vi "init.vi"(8 "error in":errorcluster, 10 "TBM module configuration in":refnum<class "TBM module configuration.lvclass">, 11 "dds runtime in":refnum<class "dds runtime.lvclass">) -> (0 "error out":errorcluster, 1 "data allocations":T1, 2 "execution settings":T4, 3 "dds runtime out":refnum<class "dds runtime.lvclass">)   [LabVIEW 2020, in "DDS runtime.lvclass"]
doc: "Provides an interface for initializing a module at runtime. While this interface performs no operations, a child should provide an override which may open any necessary references or sessions, allocate necessary memory, and perform any final configuration validataion before providing the full configuration <b>execution data</b> to the calling process."
uses:
  dds runtime.lvclass
  <vilib>/NI/Tag Bus Module Framework/module configuration/TBM module configuration.lvclass
  <vilib>/NI/Tag Bus Module Framework/runtime/execution settings.ctl
  <vilib>/NI/Tag Bus Module Framework/channel/data tables.ctl
  <vilib>/NI/Tag Bus/dictionary/data dictionary.lvclass
  <vilib>/NI/Tag Bus/dictionary table pair.ctl
  <vilib>/NI/Tag Bus/table/data table.ctl
  configuration/dds configuration.lvclass
  configuration/dds configuration.lvclass/dds configuration.ctl
  <vilib>/NI/Tag Bus Module Framework/channel/TBM channel.lvclass/TBM channel.ctl
  dds runtime.lvclass/dds runtime.ctl
  <vilib>/NI/Tag Bus/tag/Data Type.ctl
  <vilib>/NI/Tag Bus/tag/tag descriptor.lvclass/tag descriptor.ctl
  <vilib>/RTI DDS Toolkit/VIs/AdvancedCreateReader_NumDbl.vi
  <vilib>/RTI DDS Toolkit/VIs/AdvancedCreateReader_NumSgl.vi
  <vilib>/RTI DDS Toolkit/VIs/AdvancedCreateReader_NumI64.vi
  <vilib>/RTI DDS Toolkit/VIs/AdvancedCreateReader_NumI32.vi
  <vilib>/RTI DDS Toolkit/VIs/AdvancedCreateReader_NumI16.vi
  <vilib>/RTI DDS Toolkit/VIs/AdvancedCreateReader_NumI8.vi
  <vilib>/RTI DDS Toolkit/VIs/AdvancedCreateReader_NumU64.vi
  <vilib>/RTI DDS Toolkit/VIs/AdvancedCreateReader_NumU32.vi
  <vilib>/RTI DDS Toolkit/VIs/AdvancedCreateReader_NumU16.vi
  <vilib>/RTI DDS Toolkit/VIs/AdvancedCreateReader_NumU8.vi
  <vilib>/RTI DDS Toolkit/VIs/AdvancedCreateReader_Bool.vi
  <vilib>/RTI DDS Toolkit/VIs/AdvancedCreateReader_String.vi
  <vilib>/RTI DDS Toolkit/VIs/AdvancedCreateWriter_NumDbl.vi
  <vilib>/RTI DDS Toolkit/VIs/AdvancedCreateWriter_NumSgl.vi
  <vilib>/RTI DDS Toolkit/VIs/AdvancedCreateWriter_NumI64.vi
  <vilib>/RTI DDS Toolkit/VIs/AdvancedCreateWriter_NumI32.vi
  <vilib>/RTI DDS Toolkit/VIs/AdvancedCreateWriter_NumI16.vi
  <vilib>/RTI DDS Toolkit/VIs/AdvancedCreateWriter_NumI8.vi
  <vilib>/RTI DDS Toolkit/VIs/AdvancedCreateWriter_NumU64.vi
  <vilib>/RTI DDS Toolkit/VIs/AdvancedCreateWriter_NumU32.vi
  <vilib>/RTI DDS Toolkit/VIs/AdvancedCreateWriter_NumU16.vi
  <vilib>/RTI DDS Toolkit/VIs/AdvancedCreateWriter_NumU8.vi
  <vilib>/RTI DDS Toolkit/VIs/AdvancedCreateWriter_Bool.vi
  <vilib>/RTI DDS Toolkit/VIs/AdvancedCreateWriter_String.vi
  <vilib>/NI/Tag Bus Module Framework/channel/TBM channel.lvclass
  C:/Program Files (x86)/National Instruments/LabVIEW 2020/vi.lib/NI/Tag Bus/tag/tag descriptor.lvclass
  <vilib>/NI/Tag Bus Module Framework/runtime/TBM module execution interface.lvclass
  <vilib>/NI/Tag Bus/tag/tag descriptor.lvclass
  <vilib>/RTI DDS Toolkit/Library/LVDDS_library.lvlib
  <vilib>/NI/Tag Bus/tag bus.lvlib
  <vilib>/NI/Tag Bus/table/data table.lvlib
panel:
  out "Numeric":i32
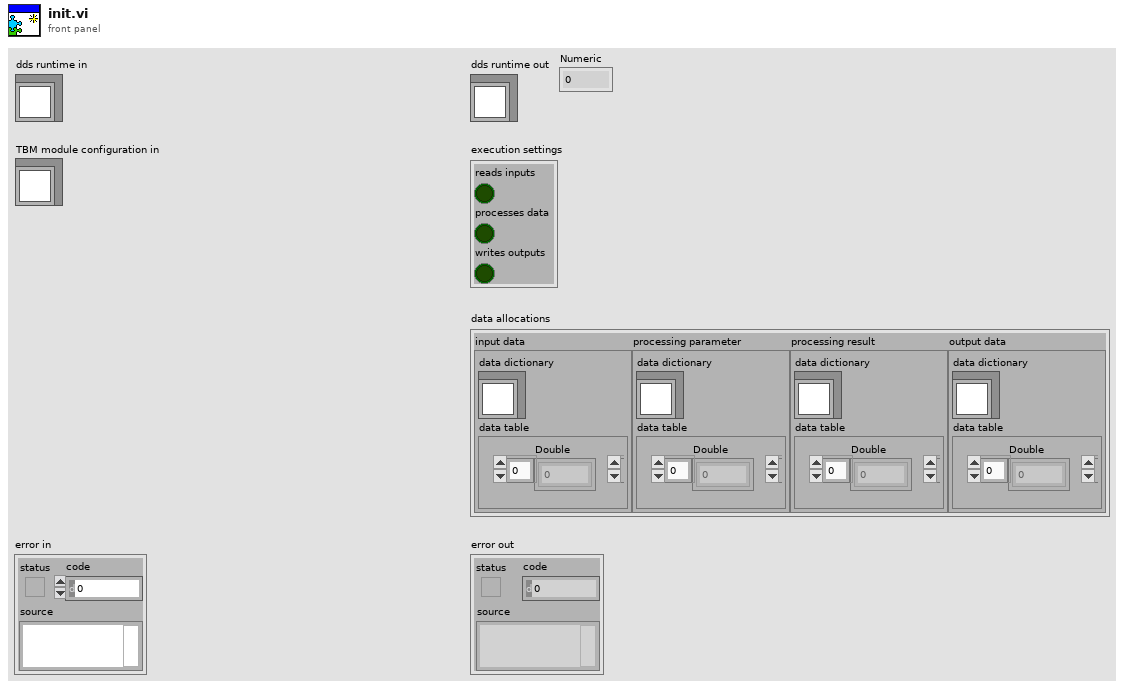
[diagram p1: front panel]
types:
  T1 = typedef "TBM channel.lvclass/data tables.ctl" = cluster{"input data":T2, "processing parameter":T2, "processing result":T2, "output data":T2}
  T2 = typedef "tag bus.lvlib/dictionary table pair.ctl" = cluster{"data dictionary":refnum<class "data dictionary.lvclass">, "data table":T3}
  T3 = typedef "tag bus.lvlib/data table.lvlib/data table.ctl" = cluster{"Double":dbl[], "Single":sgl[], "I64":i64[], "I32":i32[], "I16":i16[], "I8":i8[], "U64":u64[], "U32":u32[], "U16":u16[], "U8":u8[], "Boolean":bool[], "String":string[], "Array of Double":cluster{"DBL Array":dbl[]}[], "Array of Single":cluster{"SGL Array":sgl[]}[], "Array of I64":cluster{"I64 Array":i64[]}[], "Array of I32":cluster{"I32 Array":i32[]}[], "Array of I16":cluster{"I16 Array":i16[]}[], "Array of I8":cluster{"I8 Array":i8[]}[], "Array of U64":cluster{"U64 Array":u64[]}[], "Array of U32":cluster{"U32 Array":u32[]}[], "Array of U16":cluster{"U16 Array":u16[]}[], "Array of U8":cluster{"U8 Array":u8[]}[], "Array of Boolean":cluster{"Boolean Array":bool[]}[], "Array of String":cluster{"String Array":string[]}[]}
  T4 = typedef "TBM module execution interface.lvclass/execution settings.ctl" = cluster{"reads inputs":bool, "processes data":bool, "writes outputs":bool}
  T5 = typedef "tag bus.lvlib/tag descriptor.lvclass/Data Type.ctl" = enum16{"Double", "Single", "I64", "I32", "I16", "I8", "U64", "U32", "U16", "U8", "Boolean", "String", "Array of Double", "Array of Single", "Array of I64", "Array of I32", "Array of I16", "Array of I8", "Array of U64", "Array of U32", "Array of U16", "Array of U8", "Array of Boolean", "Array of String"}
  T6 = cluster{"index":i32, "data type":T5, "ref num":u64, "new samples only":bool, "query condition":string}
  T7 = cluster{"index":i32, "data type":T5, "ref num":u64}
  T8 = typedef "DDS configuration.lvclass/Line.ctl" = cluster{"channel":refnum<class "TBM channel.lvclass">, "DDS topic":string, "DDS Domain":u32, "advanced configuration":T9}
  T9 = typedef "LVDDS_library.lvlib/RTI DDS Advanced Reader Configuration.ctl" = cluster{"typeName":string, "keyName":string, "domainParticipantQoSProfile":string, "dataReaderQoSProfile":string, "forceArrayMapping?":bool, "forceExclusiveReader?":bool, "forceRead? (only ExclusiveReader)":bool, "forceUnboundedString?":bool}
  T10 = typedef "TBM channel.lvclass/channel classification.ctl" = enum16{"input data", "output data", "processing parameter", "processing result"}
  T11 = cluster{"index":i32, "data type":T5, "ref num":u64, "new samples only":bool, "query condition":string}[]
  T12 = cluster{"index":i32, "data type":T5, "ref num":u64}[]
  T13 = typedef "LVDDS_library.lvlib/RTI DDS Advanced Writer Configuration.ctl" = cluster{"typeName":string, "keyName":string, "domainParticipantQoSProfile":string, "dataWriterQoSProfile":string, "forceArrayMapping?":bool, "forceUnboundedString?":bool}
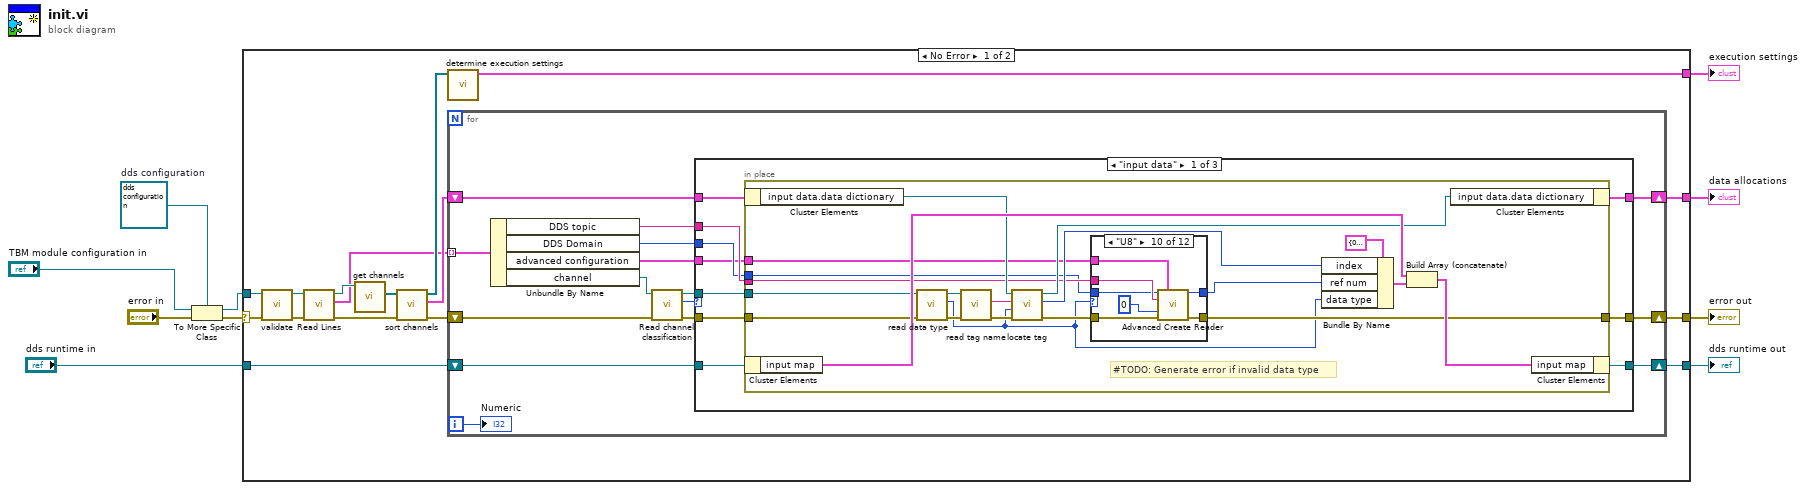
[diagram p0: block diagram]
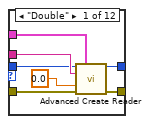
[diagram p2: hidden frame]
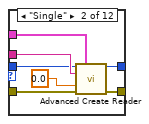
[diagram p3: hidden frame]
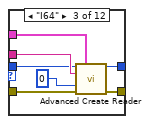
[diagram p4: hidden frame]
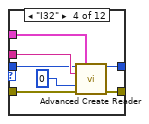
[diagram p5: hidden frame]
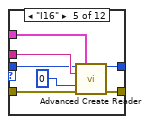
[diagram p6: hidden frame]
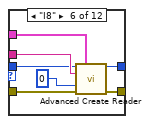
[diagram p7: hidden frame]
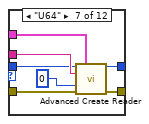
[diagram p8: hidden frame]
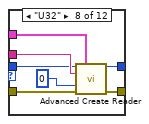
[diagram p9: hidden frame]
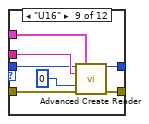
[diagram p10: hidden frame]
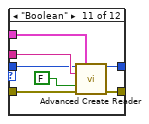
[diagram p11: hidden frame]
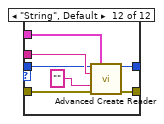
[diagram p12: hidden frame]
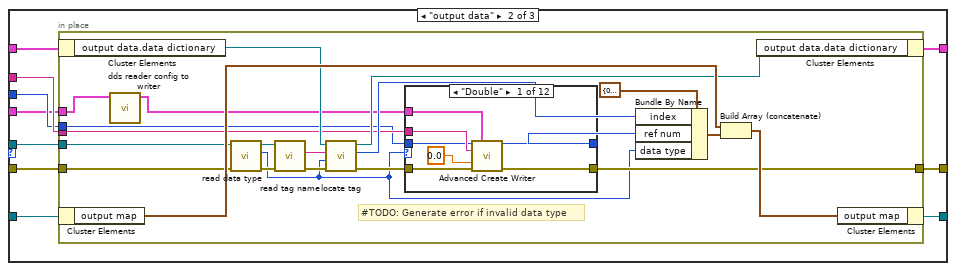
[diagram p13: hidden frame]
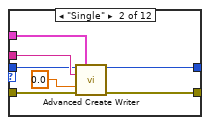
[diagram p14: hidden frame]
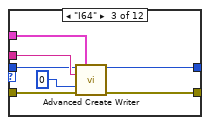
[diagram p15: hidden frame]
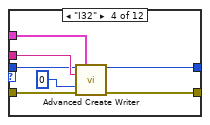
[diagram p16: hidden frame]
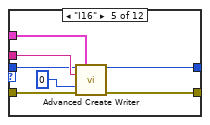
[diagram p17: hidden frame]
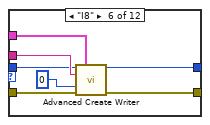
[diagram p18: hidden frame]
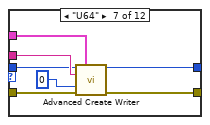
[diagram p19: hidden frame]
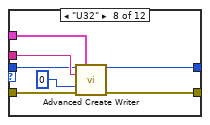
[diagram p20: hidden frame]
diagram:
  w8 = refnum<class "dds configuration.lvclass"> refnum  # dds configuration
  n1 = To More Specific Class(target class=w8, reference="TBM module configuration in", error in="error in") -> (specific class reference=w9:refnum<class "dds configuration.lvclass">, error out=w10:errorcluster)
  n2 = case shown="No Error" w10 {
    selector: w10 -> [w25 w274]
    tunnel: w9 -> [w24 _]
    tunnel: "dds runtime in" -> [w23 w275]
    tunnel: [w22 w275] -> w4
    tunnel: [w12 w274] -> w3
    tunnel: [w11 _] -> w1
    tunnel: [w26 _] -> w2
    frame No Error {
      n3 = call-dynamic "validate.vi"("error in"=w25, "dds configuration in"=w24) -> ("error out"=w17:errorcluster, "dds configuration out"=w18:refnum<class "dds configuration.lvclass">)  [unwired: 8 in]
      n4 = call "Read Lines.vi"("error in (no error)"=w17, "dds configuration in"=w18) -> ("error out"=w16:errorcluster, "Lines"=w14:T8[], "dds configuration out"=w15:refnum<class "dds configuration.lvclass">)  [unwired: 7 in]
      n5 = call-dynamic "get channels.vi"("dds configuration in"=w15) -> ("channels"=w21:refnum<class "TBM channel.lvclass">[])  [unwired: 9 in, 1 out]
      n6 = call <vilib>:"sort channels.vi"("error in"=w16, "channels in"=w21) -> ("error out"=w13:errorcluster, "data allocations"=w19:T1, "channels out"=w20:refnum<class "TBM channel.lvclass">[])  [unwired: 7 in]
      n7 = call <vilib>:"determine execution settings.vi"("channels"=w20) -> ("execution settings"=w26:T4)  [unwired: 10 in]
      n8 = for {
        shift-right: [w38] -> w22
        shift-left: w23 -> [w41]
        tunnel: w14 -> [w35] mode=indexing
        shift-right: [w30] -> w12
        shift-left: w13 -> [w31]
        shift-right: [w28] -> w11
        shift-left: w19 -> [w36]
        i -> [w27]
        n9 = Unbundle By Name(w35) -> ("DDS topic"=w34:string, "DDS Domain"=w33:u32, "advanced configuration"=w32:T9, "channel"=w29:refnum<class "TBM channel.lvclass">)
        n10 = call <vilib>:"Read channel classification.vi"("error in"=w31, "channel in"=w29) -> ("error out"=w37:errorcluster, "channel classification"=w40:T10, "channel out"=w39:refnum<class "TBM channel.lvclass">)  [unwired: 7 in]
        n11 = case shown="\"input data\"" w40 {
          tunnel: w41 -> [w51 w165 w271]
          tunnel: w39 -> [w48 w162 _]
          tunnel: [w50 w164 w271] -> w38
          tunnel: w37 -> [w49 w163 w272]
          tunnel: w36 -> [w47 w161 w273]
          tunnel: w34 -> [w46 w160 _]
          tunnel: w33 -> [w45 w159 _]
          tunnel: w32 -> [w44 w158 _]
          tunnel: [w43 w157 w272] -> w30
          tunnel: [w42 w156 w273] -> w28
          frame "input data" {
            n12 = in-place {
              in-place-border: w49 -> [w69]
              in-place-border: w48 -> [w67]
              in-place-border: w46 -> [w59]
              in-place-border: w45 -> [w58]
              in-place-border: w44 -> [w57]
              in-place-border: [w55] -> w43
              # "#TODO: Generate error if invalid data type"
              n13 = in-place-cluster #1(w47) -> ("input data.data dictionary"=w66:refnum<class "data dictionary.lvclass">)
              n14 = in-place-cluster #2(w51) -> ("input map"=w71:T11)
              n15 = call <vilib>:"read data type.vi"("error in"=w69, "system tag in"=w67) -> ("error out"=w63:errorcluster, "data type"=w53:T5, "system tag out"=w64:refnum<class "TBM channel.lvclass">)  [unwired: 7 in]
              n16 = call <vilib>:"read tag name.vi"("error in"=w63, "system tag in"=w64) -> ("error out"=w56:errorcluster, "name"=w62:string)  [unwired: 7 in, 1 out]
              n17 = call <vilib>:"locate tag.vi"("error in"=w56, "data type"=w53, "name"=w62, "data dictionary in"=w66) -> ("error out"=w61:errorcluster, "index"=w60:i32, "data dictionary out"=w65:refnum<class "data dictionary.lvclass">)  [unwired: 5 in]
              n18 = case shown="\"U8\"" w53 {
                tunnel: [w78 w85 w92 w99 w106 w113 w120 w127 w134 w141 w148 w155] -> w54
                tunnel: w61 -> [w76 w83 w90 w97 w104 w111 w118 w125 w132 w139 w146 w153]
                tunnel: [w75 w82 w89 w96 w103 w110 w117 w124 w131 w138 w145 w152] -> w55
                tunnel: w59 -> [w74 w81 w88 w95 w102 w109 w116 w123 w130 w137 w144 w151]
                tunnel: w58 -> [w73 w80 w87 w94 w101 w108 w115 w122 w129 w136 w143 w150]
                tunnel: w57 -> [w72 w79 w86 w93 w100 w107 w114 w121 w128 w135 w142 w149]
                frame "Double" {
                  n19 = call-poly <vilib>:"Advanced Create Reader.vi"("Domain Id"=w73, "Advanced Reader Configuration"=w72, "Topic Name"=w74, "Data Type"=0.0, "error in (no error)"=w76) -> ("DDS Object Ref"=w78:u64, "error out"=w75:errorcluster)  [unwired: 9 in]
                }
                frame "Single" {
                  n20 = call-poly <vilib>:"Advanced Create Reader.vi"("Domain Id"=w80, "Advanced Reader Configuration"=w79, "Topic Name"=w81, "Data Type"=sgl 0.0, "error in (no error)"=w83) -> ("DDS Object Ref"=w85:u64, "error out"=w82:errorcluster)  [unwired: 9 in]
                }
                frame "I64" {
                  n21 = call-poly <vilib>:"Advanced Create Reader.vi"("Domain Id"=w87, "Advanced Reader Configuration"=w86, "Topic Name"=w88, "Data Type"=i64 0, "error in (no error)"=w90) -> ("DDS Object Ref"=w92:u64, "error out"=w89:errorcluster)  [unwired: 9 in]
                }
                frame "I32" {
                  n22 = call-poly <vilib>:"Advanced Create Reader.vi"("Domain Id"=w94, "Advanced Reader Configuration"=w93, "Topic Name"=w95, "Data Type"=0, "error in (no error)"=w97) -> ("DDS Object Ref"=w99:u64, "error out"=w96:errorcluster)  [unwired: 9 in]
                }
                frame "I16" {
                  n23 = call-poly <vilib>:"Advanced Create Reader.vi"("Domain Id"=w101, "Advanced Reader Configuration"=w100, "Topic Name"=w102, "Data Type"=i16 0, "error in (no error)"=w104) -> ("DDS Object Ref"=w106:u64, "error out"=w103:errorcluster)  [unwired: 9 in]
                }
                frame "I8" {
                  n24 = call-poly <vilib>:"Advanced Create Reader.vi"("Domain Id"=w108, "Advanced Reader Configuration"=w107, "Topic Name"=w109, "Data Type"=i8 0, "error in (no error)"=w111) -> ("DDS Object Ref"=w113:u64, "error out"=w110:errorcluster)  [unwired: 9 in]
                }
                frame "U64" {
                  n25 = call-poly <vilib>:"Advanced Create Reader.vi"("Domain Id"=w115, "Advanced Reader Configuration"=w114, "Topic Name"=w116, "value"=u64 0, "error in (no error)"=w118) -> ("DDS Object Ref"=w120:u64, "error out"=w117:errorcluster)  [unwired: 9 in]
                }
                frame "U32" {
                  n26 = call-poly <vilib>:"Advanced Create Reader.vi"("Domain Id"=w122, "Advanced Reader Configuration"=w121, "Topic Name"=w123, "Data Type"=u32 0, "error in (no error)"=w125) -> ("DDS Object Ref"=w127:u64, "error out"=w124:errorcluster)  [unwired: 9 in]
                }
                frame "U16" {
                  n27 = call-poly <vilib>:"Advanced Create Reader.vi"("Domain Id"=w129, "Advanced Reader Configuration"=w128, "Topic Name"=w130, "Data Type"=u16 0, "error in (no error)"=w132) -> ("DDS Object Ref"=w134:u64, "error out"=w131:errorcluster)  [unwired: 9 in]
                }
                frame "U8" {
                  n28 = call-poly <vilib>:"Advanced Create Reader.vi"("Domain Id"=w136, "Advanced Reader Configuration"=w135, "Topic Name"=w137, "Data Type"=u8 0, "error in (no error)"=w139) -> ("DDS Object Ref"=w141:u64, "error out"=w138:errorcluster)  [unwired: 9 in]
                }
                frame "Boolean" {
                  n29 = call-poly <vilib>:"Advanced Create Reader.vi"("Domain Id"=w143, "Advanced Reader Configuration"=w142, "Topic Name"=w144, "Data Type"=FALSE, "error in (no error)"=w146) -> ("DDS Object Ref"=w148:u64, "error out"=w145:errorcluster)  [unwired: 9 in]
                }
                frame "String", Default {
                  n30 = call-poly <vilib>:"Advanced Create Reader.vi"("Domain Id"=w150, "Advanced Reader Configuration"=w149, "Topic Name"=w151, "Data Type"="", "error in (no error)"=w153) -> ("DDS Object Ref"=w155:u64, "error out"=w152:errorcluster)  [unwired: 9 in]
                }
              }
              n31 = Bundle By Name(cluster=T6 {"index"=0, "data type"=enum."Double", "ref num"=0, "new samples only"=FALSE, "query condition"=""} ("item"), "index"=w60, "ref num"=w54, "data type"=w53) -> (w68:T6)
              n32 = Build Array (concatenate)(w71, w68) -> (w70:T11)
              n33 = in-place-cluster #1("input data.data dictionary"=w65) -> (w42:T1)
              n34 = in-place-cluster #2("input map"=w70) -> (w50:refnum<class "dds runtime.lvclass">)
            }
          }
          frame "output data" {
            n35 = in-place {
              in-place-border: w163 -> [w184]
              in-place-border: w162 -> [w181]
              in-place-border: w160 -> [w173]
              in-place-border: w159 -> [w172]
              in-place-border: w158 -> [w167]
              in-place-border: [w170] -> w157
              # "#TODO: Generate error if invalid data type"
              n36 = in-place-cluster #3(w161) -> ("output data.data dictionary"=w180:refnum<class "data dictionary.lvclass">)
              n37 = in-place-cluster #4(w165) -> ("output map"=w186:T12)
              n38 = call "dds reader config to writer.vi"("reader configuration"=w167) -> ("writer configuration"=w166:T13)  [unwired: 10 in]
              n39 = call <vilib>:"read data type.vi"("error in"=w184, "system tag in"=w181) -> ("error out"=w177:errorcluster, "data type"=w168:T5, "system tag out"=w178:refnum<class "TBM channel.lvclass">)  [unwired: 7 in]
              n40 = call <vilib>:"read tag name.vi"("error in"=w177, "system tag in"=w178) -> ("error out"=w171:errorcluster, "name"=w176:string)  [unwired: 7 in, 1 out]
              n41 = call <vilib>:"locate tag.vi"("error in"=w171, "data type"=w168, "name"=w176, "data dictionary in"=w180) -> ("error out"=w175:errorcluster, "index"=w174:i32, "data dictionary out"=w179:refnum<class "data dictionary.lvclass">)  [unwired: 5 in]
              n42 = case shown="\"Double\"" w168 {
                tunnel: [w193 w200 w207 w214 w221 w228 w235 w242 w249 w256 w263 w270] -> w169
                tunnel: w175 -> [w191 w198 w205 w212 w219 w226 w233 w240 w247 w254 w261 w268]
                tunnel: [w190 w197 w204 w211 w218 w225 w232 w239 w246 w253 w260 w267] -> w170
                tunnel: w173 -> [w189 w196 w203 w210 w217 w224 w231 w238 w245 w252 w259 w266]
                tunnel: w172 -> [w188 w195 w202 w209 w216 w223 w230 w237 w244 w251 w258 w265]
                tunnel: w166 -> [w187 w194 w201 w208 w215 w222 w229 w236 w243 w250 w257 w264]
                frame "Double" {
                  n43 = call-poly <vilib>:"Advanced Create Writer.vi"("Domain Id"=w188, "Advanced Writer Configuration"=w187, "Topic Name"=w189, "Data Type"=0.0, "error in (no error)"=w191) -> ("DDS Object Ref"=w193:u64, "error out"=w190:errorcluster)  [unwired: 9 in]
                }
                frame "Single" {
                  n44 = call-poly <vilib>:"Advanced Create Writer.vi"("Domain Id"=w195, "Advanced Writer Configuration"=w194, "Topic Name"=w196, "Data Type"=sgl 0.0, "error in (no error)"=w198) -> ("DDS Object Ref"=w200:u64, "error out"=w197:errorcluster)  [unwired: 9 in]
                }
                frame "I64" {
                  n45 = call-poly <vilib>:"Advanced Create Writer.vi"("Domain Id"=w202, "Advanced Writer Configuration"=w201, "Topic Name"=w203, "Data Type"=i64 0, "error in (no error)"=w205) -> ("DDS Object Ref"=w207:u64, "error out"=w204:errorcluster)  [unwired: 9 in]
                }
                frame "I32" {
                  n46 = call-poly <vilib>:"Advanced Create Writer.vi"("Domain Id"=w209, "Advanced Writer Configuration"=w208, "Topic Name"=w210, "Data Type"=0, "error in (no error)"=w212) -> ("DDS Object Ref"=w214:u64, "error out"=w211:errorcluster)  [unwired: 9 in]
                }
                frame "I16" {
                  n47 = call-poly <vilib>:"Advanced Create Writer.vi"("Domain Id"=w216, "Advanced Writer Configuration"=w215, "Topic Name"=w217, "Data Type"=i16 0, "error in (no error)"=w219) -> ("DDS Object Ref"=w221:u64, "error out"=w218:errorcluster)  [unwired: 9 in]
                }
                frame "I8" {
                  n48 = call-poly <vilib>:"Advanced Create Writer.vi"("Domain Id"=w223, "Advanced Writer Configuration"=w222, "Topic Name"=w224, "Data Type"=i8 0, "error in (no error)"=w226) -> ("DDS Object Ref"=w228:u64, "error out"=w225:errorcluster)  [unwired: 9 in]
                }
                frame "U64" {
                  n49 = call-poly <vilib>:"Advanced Create Writer.vi"("Domain Id"=w230, "Advanced Writer Configuration"=w229, "Topic Name"=w231, "Data Type"=u64 0, "error in (no error)"=w233) -> ("DDS Object Ref"=w235:u64, "error out"=w232:errorcluster)  [unwired: 9 in]
                }
                frame "U32" {
                  n50 = call-poly <vilib>:"Advanced Create Writer.vi"("Domain Id"=w237, "Advanced Writer Configuration"=w236, "Topic Name"=w238, "Data Type"=u32 0, "error in (no error)"=w240) -> ("DDS Object Ref"=w242:u64, "error out"=w239:errorcluster)  [unwired: 9 in]
                }
                frame "U16" {
                  n51 = call-poly <vilib>:"Advanced Create Writer.vi"("Domain Id"=w244, "Advanced Writer Configuration"=w243, "Topic Name"=w245, "Data Type"=u16 0, "error in (no error)"=w247) -> ("DDS Object Ref"=w249:u64, "error out"=w246:errorcluster)  [unwired: 9 in]
                }
                frame "U8" {
                  n52 = call-poly <vilib>:"Advanced Create Writer.vi"("Domain Id"=w251, "Advanced Writer Configuration"=w250, "Topic Name"=w252, "Data Type"=u8 0, "error in (no error)"=w254) -> ("DDS Object Ref"=w256:u64, "error out"=w253:errorcluster)  [unwired: 9 in]
                }
                frame "Boolean" {
                  n53 = call-poly <vilib>:"Advanced Create Writer.vi"("Domain Id"=w258, "Advanced Writer Configuration"=w257, "Topic Name"=w259, "Data Type"=FALSE, "error in (no error)"=w261) -> ("DDS Object Ref"=w263:u64, "error out"=w260:errorcluster)  [unwired: 9 in]
                }
                frame "String", Default {
                  n54 = call-poly <vilib>:"Advanced Create Writer.vi"("Domain Id"=w265, "Advanced Writer Configuration"=w264, "Topic Name"=w266, "Data Type"="", "error in (no error)"=w268) -> ("DDS Object Ref"=w270:u64, "error out"=w267:errorcluster)  [unwired: 9 in]
                }
              }
              n55 = Bundle By Name(cluster=T7 {"index"=0, "data type"=enum."Double", "ref num"=0} ("item"), "index"=w174, "ref num"=w169, "data type"=w168) -> (w182:T7)
              n56 = Build Array (concatenate)(w186, w182) -> (w185:T12)
              n57 = in-place-cluster #3("output data.data dictionary"=w179) -> (w156:T1)
              n58 = in-place-cluster #4("output map"=w185) -> (w164:refnum<class "dds runtime.lvclass">)
            }
          }
          frame Default {
          }
        }
        "Numeric" <- w27
      }
    }
    frame Error {
    }
  }
  "error out" <- w3
  "dds runtime out" <- w4
  "execution settings" <- w2
  "data allocations" <- w1
